vi "UI.Addon.Path.Parse.vi"(11 "Cached Addon Path":string) -> (0 "Addon Name":string, 1 "IP Address":string, 2 "Controller and IP Address":string, 3 "Addon Path":string, 4 "Remaining Path":string)   [LabVIEW 2019, in "Control Workspace Shared.lvlib"]
uses:
  Control Workspace Shared.lvlib
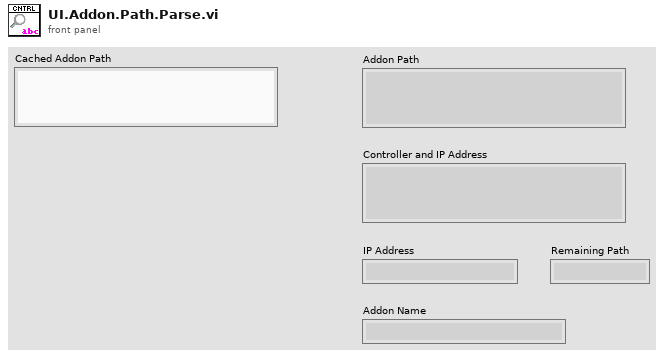
[diagram p1: front panel]
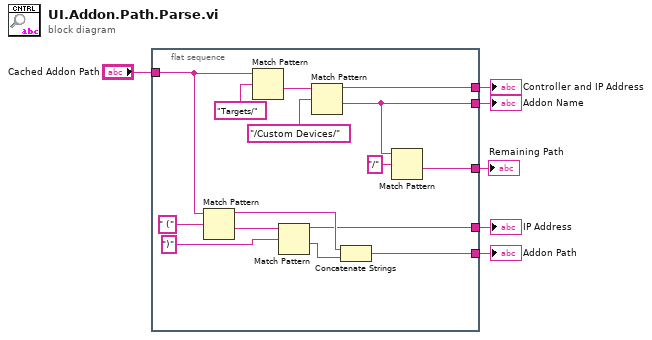
[diagram p0: block diagram]
diagram:
  n1 = flat-sequence {
    tunnel: [w15] -> w3
    tunnel: "Cached Addon Path" -> [w10]
    tunnel: [w17] -> w5
    tunnel: [w11] -> w6
    tunnel: [w9] -> w2
    tunnel: [w7] -> w1
    frame #0 {
      n2 = Match Pattern(string=w10, regular expression=" (") -> (before substring=w18:string, after substring=w19:string)  [unwired: 1 in, 2 out]
      n3 = Match Pattern(string=w10, regular expression="Targets/") -> (after substring=w12:string)  [unwired: 1 in, 3 out]
      n4 = Match Pattern(string=w19, regular expression=")") -> (before substring=w15:string, after substring=w14:string)  [unwired: 1 in, 2 out]
      n5 = Match Pattern(string=w12, regular expression="/Custom Devices/") -> (before substring=w11:string, after substring=w9:string)  [unwired: 1 in, 2 out]
      n6 = Concatenate Strings(w18, w14) -> (w17:string)
      n7 = Match Pattern(string=w9, regular expression="/") -> (after substring=w7:string)  [unwired: 1 in, 3 out]
    }
  }
  "Controller and IP Address" <- w6
  "Addon Path" <- w5
  "IP Address" <- w3
  "Addon Name" <- w2
  "Remaining Path" <- w1
